vi "Add Color in OneRow.vi"(8 "error in (no error)":errorcluster, 10 "1 Row Data":string[](array[string]), 11 "MCLB_Lib in":refnum<class "MCLB_Lib.lvclass">) -> (0 "error out":errorcluster, 3 "MCLB_Lib out":refnum<class "MCLB_Lib.lvclass">)   [LabVIEW 2021, in "MCLB_Lib.lvclass"]
uses:
  <userlib>/John_Lib/MCLB/MCLB_Lib.lvclass
  <userlib>/John_Lib/MCLB/MCLB_Lib.lvclass/MCLB_Lib.ctl
  4be8bae2-d552-47f9-8b02-75517a057aec.vi
  <vilib>/Utility/miscctls.llb/LVRowAndColumnTypeDef.ctl
  de0307f1-042a-4276-a304-54001a54e947.vi
  d75f7507-2910-489f-9562-1086008e6bb9.vi
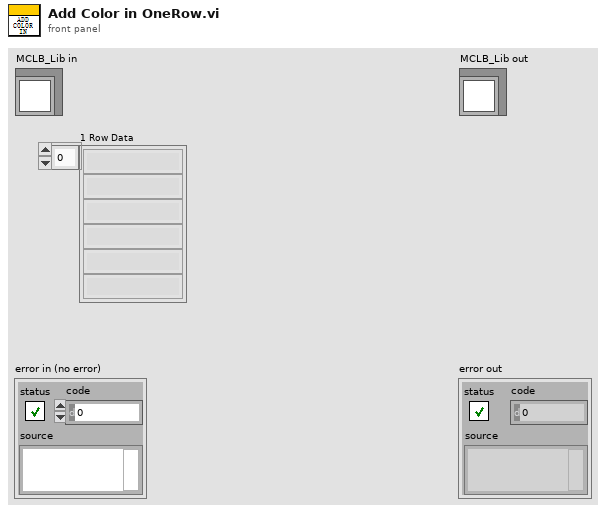
[diagram p1: front panel]
types:
  T1 = typedef "LVRowAndColumnTypeDef.ctl" = cluster{"Row":i32, "Column":i32}
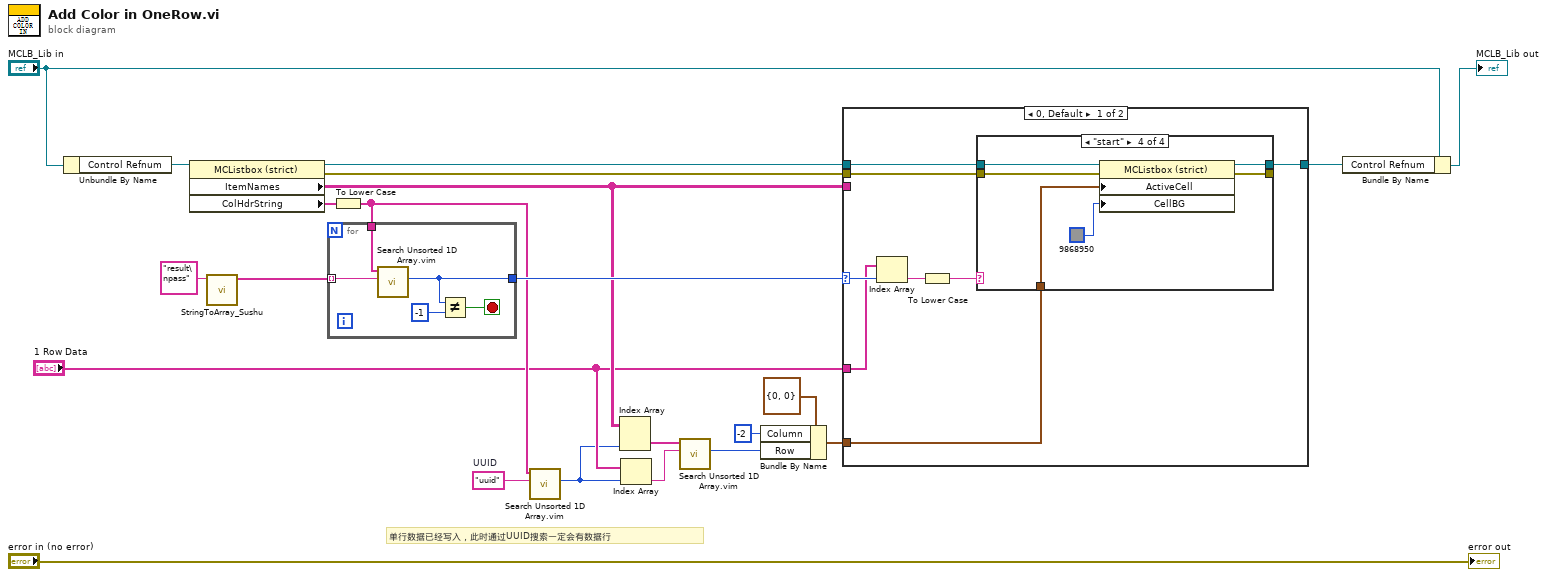
[diagram p0: block diagram]
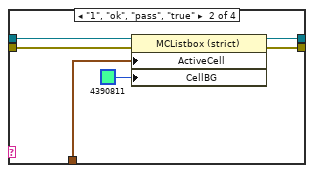
[diagram p3: hidden frame]
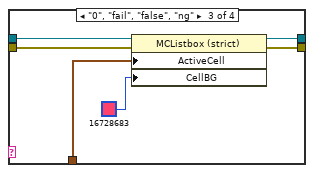
[diagram p4: hidden frame]
diagram:
  w12 = "uuid"  # UUID
  # "单行数据已经写入，此时通过UUID搜索一定会有数据行"
  n1 = Unbundle By Name("MCLB_Lib in") -> ("Control Refnum"=w18:refnum<vi>)
  n2 = property class="MCListbox (strict)"(reference=w18) -> (reference out=w20:refnum<vi>, error out=w21:errorcluster, "ItemNames"=w4:string[][], "ColHdrString"=w11:string[])  [unwired: 1 in]
  n3 = call <userlib>:"StringToArray_Sushu.vi"("State Queue"="result\npass") -> ("Array"=w16:string[])  [unwired: 7 in, 3 out]
  n4 = To Lower Case(string=w11) -> (all lower case string=w7:string[])
  n5 = for {
    tunnel: [w25] -> w19
    tunnel: w7 -> [w27]
    tunnel: w16 -> [w26] mode=indexing
    stop <- w23 stop-if-true
    n6 = call "Search Unsorted 1D Array.vim"("element"=w26, "unsorted 1D array"=w27) -> ("index of element"=w25:i32)  [unwired: 9 in]
    n7 = Not Equal?(x=w25, y=-1) -> (x != y?=w23:bool)
  }
  n8 = call "Search Unsorted 1D Array.vim"("element"=w12, "unsorted 1D array"=w7) -> ("index of element"=w2:i32)  [unwired: 9 in]
  n9 = Index Array(array=w4, index (col)=w2) -> (element=w5:string[])  [unwired: 1 in]
  n10 = Index Array(array="1 Row Data", index=w2) -> (element=w6:string)
  n11 = call "Search Unsorted 1D Array.vim"("element"=w6, "unsorted 1D array"=w5) -> ("index of element"=w1:i32)  [unwired: 9 in]
  n12 = Bundle By Name(cluster=T1 {"Row"=0, "Column"=0} ("Active Cell:Active Cell"), "Column"=-2, "Row"=w1) -> (w14:T1)
  n13 = case shown="0, Default" w19 {
    selector: w19 -> [w35 _]
    tunnel: "1 Row Data" -> [w34 _]
    tunnel: w4 -> [_ _]
    tunnel: [w29 w56] -> w10
    tunnel: w20 -> [w33 w56]
    tunnel: w21 -> [w32 _]
    tunnel: w14 -> [w30 _]
    frame 0, Default {
      n14 = Index Array(array=w34, index=w35) -> (element=w31:string)
      n15 = To Lower Case(string=w31) -> (all lower case string=w28:string)
      n16 = case shown="\"start\"" w28 {
        tunnel: w33 -> [w37 w43 w49 w55]
        tunnel: [w37 w42 w48 w54] -> w29
        tunnel: w32 -> [w36 w41 w47 w53]
        tunnel: [w36 w40 w46 w52] -> _
        tunnel: w30 -> [_ w38 w44 w50]
        frame Default {
        }
        frame "1", "ok", "pass", "true" {
          n17 = property on="Property Node" class="MCListbox (strict)"(reference=w43, error in=w41, "ActiveCell"=w38, "CellBG"=u32 4390811 ("Color Box 2")) -> (reference out=w42:refnum<vi>, error out=w40:errorcluster)
        }
        frame "0", "fail", "false", "ng" {
          n18 = property on="Property Node" class="MCListbox (strict)"(reference=w49, error in=w47, "ActiveCell"=w44, "CellBG"=u32 16728683 ("Color Box 2")) -> (reference out=w48:refnum<vi>, error out=w46:errorcluster)
        }
        frame "start" {
          n19 = property on="Property Node" class="MCListbox (strict)"(reference=w55, error in=w53, "ActiveCell"=w50, "CellBG"=u32 9868950 ("Color Box 2")) -> (reference out=w54:refnum<vi>, error out=w52:errorcluster)
        }
      }
    }
    frame -1 {
      # "无结果列，不添加颜色"
    }
  }
  n20 = Bundle By Name(cluster="MCLB_Lib in", "Control Refnum"=w10) -> (→"MCLB_Lib out":refnum<class "MCLB_Lib.lvclass">)
  "error out" <- "error in (no error)"
